vi "Main.vi"() -> ()   [LabVIEW 2013]
uses:
  src/LabVIEW/Qt Widgets/LQWidgetEngine/LQWidgetEngine.lvclass
  src/LabVIEW/LQ Core/Qt/Orientation.ctl
  src/LabVIEW/LQ Core/Qt/AlignmentFlag.ctl
  src/LabVIEW/LQ Core/QSize.ctl
  src/LabVIEW/Qt Widgets/QBoxLayout/Direction.ctl
  src/LabVIEW/LQ Core/LQCoreEngine/_Polymorphic Instances/Connect_EventRefOut_DBL.vi
  src/LabVIEW/Qt Widgets/QScrollArea/setAlignment.vi
  src/LabVIEW/Qwt/QwtAbstractScale/setUpperBound.vi
  src/LabVIEW/Qwt/QwtAbstractScale/setScaleStepSize.vi
  src/LabVIEW/Qwt/QwtAbstractSlider/setValue.vi
  src/LabVIEW/Qt Widgets/QWidget/resize.vi
  src/LabVIEW/Qt Widgets/QWidget/setVisible.vi
  src/LabVIEW/Qt GUI/LQGuiEngine/setWindowIcon.vi
  src/LabVIEW/Qt Widgets/QWidget/sizeHint.vi
  src/LabVIEW/LQ Core/LQCoreEngine/LQCoreEngine.lvclass
  src/LabVIEW/Qt Widgets/QBoxLayout/QBoxLayout.lvclass
  src/LabVIEW/Qwt/QwtSlider/QwtSlider.lvclass
  src/LabVIEW/LQ Core/Qt/Qt.lvlib
  src/LabVIEW/Qt SVG/QSvgWidget/QSvgWidget.lvclass
  src/LabVIEW/Qt GUI/QIcon/QIcon.lvclass
  src/LabVIEW/Qt Widgets/QScrollArea/QScrollArea.lvclass
  src/LabVIEW/Qt Widgets/QWidget/QWidget.lvclass
panel:
  in  "Stop Button":bool
  # "Prerequisite knowledge/experience\n- Basic LabVIEW programming\n- Example 3b. Connecting a Signal to a LabVIEW Event from the \"Hello World - Introduction to Widgets\"\n   series\n\n\nDescription\nThis example displays an SVG image and lets you change its magnification, to demonstrate the\nsmoothness of vector graphics at different zoom levels. It also showcases a user-defined scroll area,\nwhich is useful for containing a scene that is too large to fit on the screen (e.g. an SVG image that's\nmagnified 20x).\n\n\nShowcase\n- SVG rendering\n- User-defined scroll area"
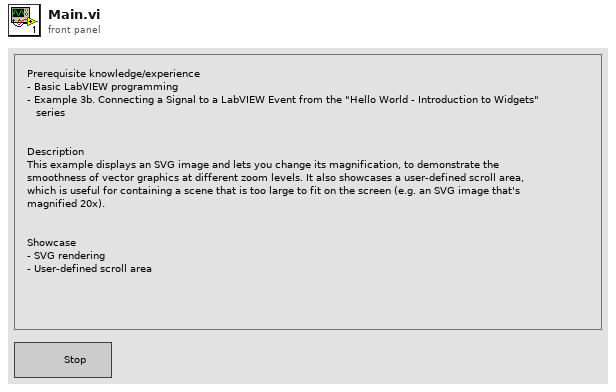
[diagram p1: front panel]
types:
  T1 = typedef "QBoxLayout.lvclass/Direction.ctl" = i32
  T2 = typedef "QSize.ctl" = cluster{"width":i32, "height":i32}
  T3 = typedef "Qt.lvlib/AlignmentFlag.ctl" = i32
  T4 = typedef "Qt.lvlib/Orientation.ctl" = i32
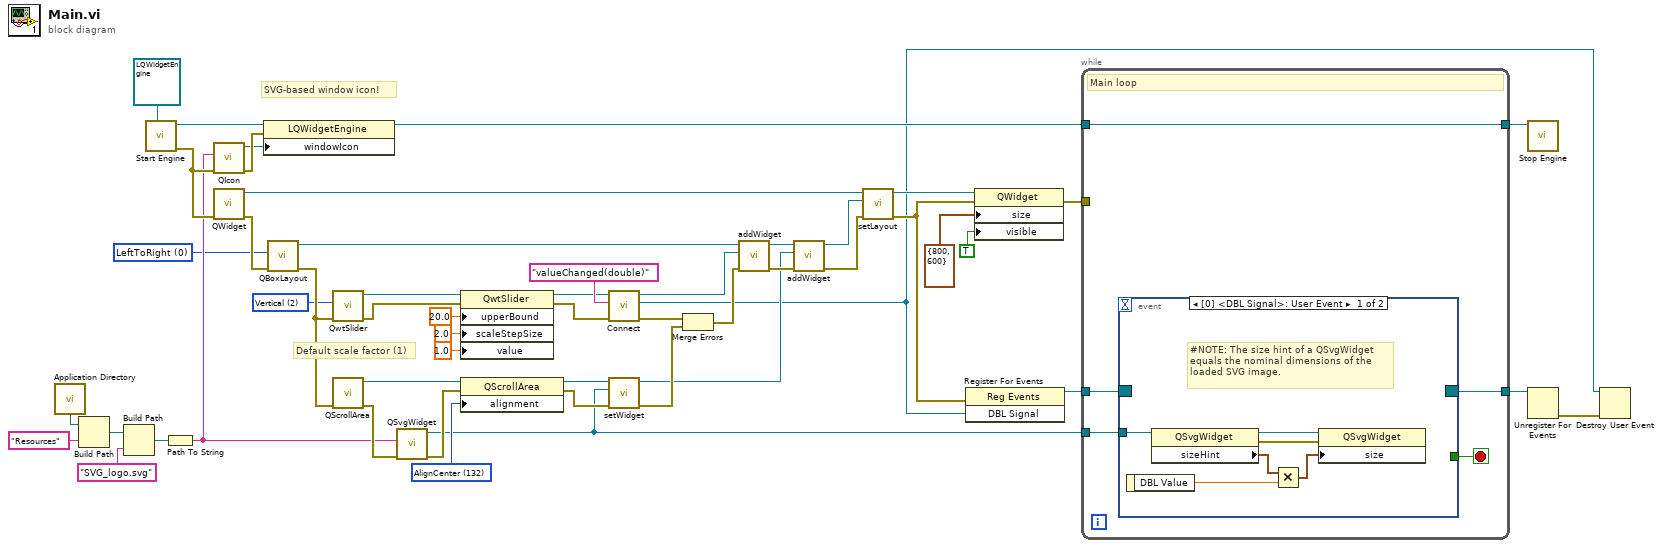
[diagram p0: block diagram]
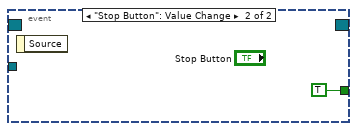
[diagram p2: hidden frame]
diagram:
  w6 = T1 0 items=["LeftToRight", "RightToLeft", "TopToBottom", "BottomToTop"] ("direction")
  w31 = T3 132 items=["AlignLeading"=1, "AlignTrailing"=2, "AlignHCenter"=4, "AlignJustify"=8, "AlignAbsolute"=16, "AlignHorizontal_Mask"=31, "AlignTop"=32, "AlignBottom"=64, "AlignVCenter"=128, "AlignBaseline"=256, "AlignVertical_Mask"=480, "AlignCenter"=132] ("alignment")
  w41 = T4 2 items=["Horizontal"=1, "Vertical"=2] ("orientation")
  # "Default scale factor (1)"
  # "SVG-based window icon!"
  n1 = call <vilib>:"Application Directory.vi"() -> ("Application Directory"=w39:path)
  n2 = Build Path(base path=w39, name or relative path="Resources") -> (appended path=w37:path)
  n3 = Build Path(base path=w37, name or relative path="SVG_logo.svg" ("fileName")) -> (appended path=w36:path)
  n4 = call "Start Engine.vi"("Engine Type"=refnum<class "LQWidgetEngine.lvclass"> refnum ("Qt Widgets.lvlib:LQWidgetEngine")) -> ("Error Out"=w45:errorcluster, "New Engine"=w40:refnum<class "LQWidgetEngine.lvclass">)  [unwired: 9 in]
  n5 = Path To String(path=w36) -> (string=w35:string)
  n6 = call "QIcon.vi"("Error In"=w45, "fileName"=w35) -> ("Error Out"=w44:errorcluster, "New QIcon"=w33:refnum<class "QIcon.lvclass">)  [unwired: 8 in]
  n7 = call "QWidget.vi"("Error In"=w45) -> ("Error Out"=w46:errorcluster, "New QWidget"=w24:refnum<class "QWidget.lvclass">)  [unwired: 9 in]
  n8 = property class="LQWidgetEngine"(reference=w40, error in=w44, "windowIcon"=w33) -> (reference out=w19:refnum<class "LQWidgetEngine.lvclass">)  [unwired: 1 out]
  n9 = call "QBoxLayout.vi"("Error In"=w46, "direction"=w6) -> ("Error Out"=w47:errorcluster, "New QBoxLayout"=w28:refnum<class "QBoxLayout.lvclass">)  [unwired: 8 in]
  n10 = call "QwtSlider.vi"("Error In"=w47, "orientation"=w41) -> ("Error Out"=w5:errorcluster, "New QwtSlider"=w13:refnum<class "QwtSlider.lvclass">)  [unwired: 8 in]
  n11 = call "QScrollArea.vi"("Error In"=w47) -> ("Error Out"=w48:errorcluster, "New QScrollArea"=w32:refnum<class "QScrollArea.lvclass">)  [unwired: 9 in]
  n12 = call "QSvgWidget.vi"("Error In"=w48, "file"=w35) -> ("Error Out"=w43:errorcluster, "New QSvgWidget"=w18:refnum<class "QSvgWidget.lvclass">)  [unwired: 8 in]
  n13 = property class="QwtSlider"(reference=w13, error in=w5, "upperBound"=20.0, "scaleStepSize"=2.0 ("value"), "value"=1.0 ("scaleStepSize")) -> (reference out=w12:refnum<class "QwtSlider.lvclass">, error out=w4:errorcluster)
  n14 = property class="QScrollArea"(reference=w32, error in=w43, "alignment"=w31) -> (reference out=w30:refnum<class "QScrollArea.lvclass">, error out=w29:errorcluster)
  n15 = call-poly "Connect.vi"("Error In"=w4, "Signal Signature"="valueChanged(double)", "Sender In"=w12) -> ("Error Out"=w3:errorcluster, "DBL Signal"=w16:refnum<user-event>, "Sender Out"=w14:refnum<class "QwtSlider.lvclass">)  [unwired: 6 in]
  n16 = call "setWidget.vi"("Error In"=w29, "widget"=w18, "QScrollArea In"=w30) -> ("Error Out"=w49:errorcluster, "QScrollArea Out"=w26:refnum<class "QScrollArea.lvclass">)  [unwired: 7 in]
  n17 = Merge Errors(w3, w49) -> (w50:errorcluster)
  n18 = call "addWidget.vi"("Error In"=w50, "widget"=w14, "QBoxLayout In"=w28) -> ("Error Out"=w51:errorcluster, "QBoxLayout Out"=w27:refnum<class "QBoxLayout.lvclass">)  [unwired: 7 in]
  n19 = call "addWidget.vi"("Error In"=w51, "widget"=w26, "QBoxLayout In"=w27) -> ("Error Out"=w2:errorcluster, "QBoxLayout Out"=w23:refnum<class "QBoxLayout.lvclass">)  [unwired: 7 in]
  n20 = call "setLayout.vi"("Error In"=w2, "layout"=w23, "QWidget In"=w24) -> ("Error Out"=w52:errorcluster, "QWidget Out"=w22:refnum<class "QWidget.lvclass">)  [unwired: 7 in]
  n21 = register-events(error in=w52, w16) -> (reference out=w21:refnum<event-registration>)  [unwired: 1 in, 1 out]
  n22 = property class="QWidget"(reference=w22, error in=w52, "size"=T2 {"width"=800, "height"=600} ("minimumSize"), "visible"=TRUE) -> (error out=w1:errorcluster)  [unwired: 1 out]
  n23 = while {
    tunnel: w21 -> [w57]
    tunnel: [w56] -> w20
    tunnel: w19 -> [w56]
    tunnel: w18 -> [w54]
    tunnel: [w53] -> w17
    tunnel: w1 -> [_]
    stop <- w55 stop-if-true
    # "Main loop"
    n24 = event shown="[0] <DBL Signal>: User Event" {
      selector: w57 -> [_ _]
      dyn-events: [_ _] -> w53
      timeout: _ -> [_ _]
      tunnel: [_ TRUE] -> w55
      tunnel: w54 -> [w63 _]
      event User Event {
        # "#NOTE: The size hint of a QSvgWidget\nequals the nominal dimensions of the\nloaded SVG image."
        n25 = event-data() -> ("DBL Value"=w61:dbl)  [unwired: 1 in]
        n26 = property class="QSvgWidget"(reference=w63) -> (reference out=w62:refnum<class "QSvgWidget.lvclass">, error out=w58:errorcluster, "sizeHint"=w60:T2)  [unwired: 1 in]
        n27 = Multiply(x=w60, y=w61) -> (x*y=w59:cluster{"width":dbl, "height":dbl})
        n28 = property class="QSvgWidget"(reference=w62, error in=w58, "size"=w59) -> ()  [unwired: 2 out]
      }
      event "Stop Button": Value Change {
        n29 = event-data() -> ()  [unwired: 1 in, 1 out]
      }
    }
  }
  n30 = call "Stop Engine.vi"("LQCoreEngine"=w20) -> ()  [unwired: 10 in, 1 out]
  n31 = Unregister For Events(event registration refnum=w17) -> (error out=w15:errorcluster)  [unwired: 1 in]
  n32 = Destroy User Event(user event=w16, error in=w15) -> ()  [unwired: 1 out]
